vi "SQL删除.vi"(0 "computer1":string, 1 "ADODB._Connection In":refnum<k7>, 5 "computer2":string, 7 "computer3":string, 11 "error in (no error)":errorcluster caption="错误输入（无错误）") -> (15 "error out":errorcluster caption="错误输出")   [LabVIEW 2017]
panel:
  out "ADODB._Connection Out":refnum<k7>
  out "连接的字符串 3":string
  out "连接的字符串 2":string
  out "连接的字符串":string
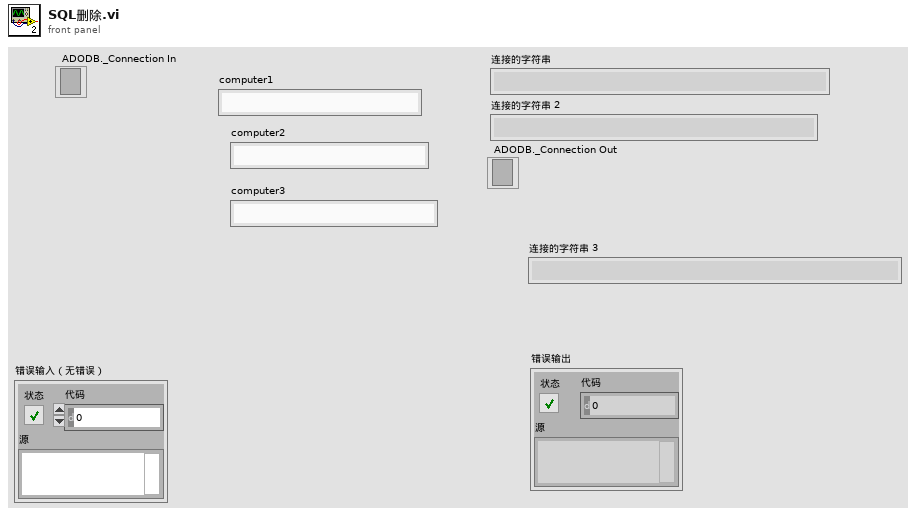
[diagram p1: front panel]
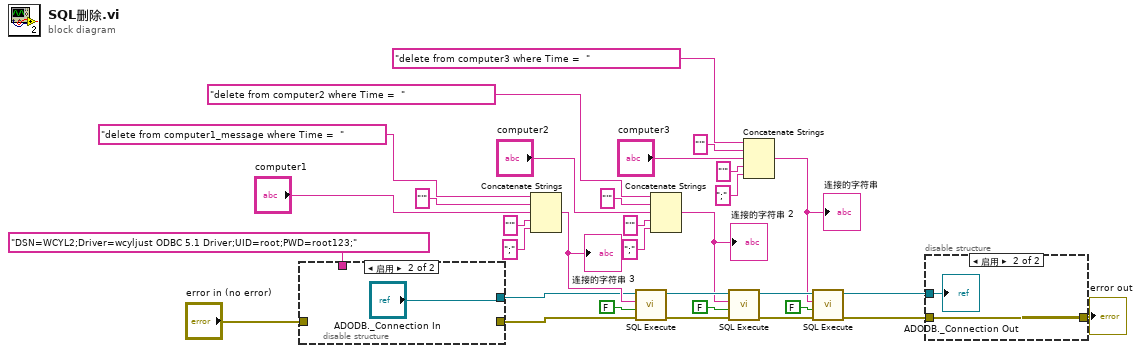
[diagram p0: block diagram]
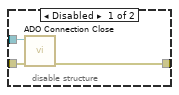
[diagram p2: hidden frame]
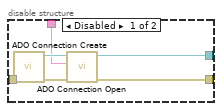
[diagram p3: hidden frame]
diagram:
  n1 = disable-structure shown="启用" {
    disable-tunnel: "DSN=WCYL2;Driver=wcyljust ODBC 5.1 Driver;UID=root;PWD=root123;" ("ConnectionString") -> [w36 _]
    disable-tunnel: "error in (no error)" -> [w35 _]
    disable-tunnel: [w34 "ADODB._Connection In"] -> w22
    disable-tunnel: [w33 _] -> w21
    frame Disabled {
      n2 = call <userlib>:"ADO Connection Create.vi"("error in (no error)"=w35) -> ("error out"=w37:errorcluster, "ADODB._Connection Out"=w38:refnum<k7>)  [unwired: 9 in]
      n3 = call <userlib>:"ADO Connection Open.vi"("error in (no error)"=w37, "ConnectionString"=w36, "ADODB._Connection In"=w38) -> ("error out"=w33:errorcluster, "ADODB._Connection Out"=w34:refnum<k7>)  [unwired: 7 in]
    }
    frame Enabled {
    }
  }
  n4 = Concatenate Strings("delete from computer1_message where Time =  " ("Command Text"), "'" ("字符串"), "computer1", "'" ("字符串"), ";" ("字符串")) -> (w28:string)
  "连接的字符串 3" <- w28
  n5 = call <userlib>:"SQL Execute.vi"("error in (no error)"=w21, "Return Data (T)"=FALSE, "Command Text"=w28, "ADODB._Connection In"=w22) -> ("error out"=w18:errorcluster, "ADODB._Connection Out"=w13:refnum<k7>)  [unwired: 4 in, 2 out]
  n6 = Concatenate Strings("delete from computer2 where Time =  " ("Command Text"), "'" ("字符串"), "computer2", "'" ("字符串"), ";" ("字符串")) -> (w2:string)
  "连接的字符串 2" <- w2
  n7 = call <userlib>:"SQL Execute.vi"("error in (no error)"=w18, "Return Data (T)"=FALSE, "Command Text"=w2, "ADODB._Connection In"=w13) -> ("error out"=w17:errorcluster, "ADODB._Connection Out"=w14:refnum<k7>)  [unwired: 4 in, 2 out]
  n8 = Concatenate Strings("delete from computer3 where Time =  " ("Command Text"), "'" ("字符串"), "computer3", "'" ("字符串"), ";" ("字符串")) -> (w1:string)
  "连接的字符串" <- w1
  n9 = call <userlib>:"SQL Execute.vi"("error in (no error)"=w17, "Return Data (T)"=FALSE, "Command Text"=w1, "ADODB._Connection In"=w14) -> ("error out"=w16:errorcluster, "ADODB._Connection Out"=w15:refnum<k7>)  [unwired: 4 in, 2 out]
  n10 = disable-structure shown="启用" {
    disable-tunnel: [w42 w44] -> w24
    disable-tunnel: w16 -> [w41 w44]
    disable-tunnel: w15 -> [w40 w43]
    frame Disabled {
      n11 = call <userlib>:"ADO Connection Close.vi"("error in (no error)"=w41, "ADODB._Connection In"=w40) -> ("error out"=w42:errorcluster)  [unwired: 8 in, 1 out]
    }
    frame Enabled {
      "ADODB._Connection Out" <- w43
    }
  }
  "error out" <- w24
